vi "GetActiveFieldName.vi"(1 "protobuf index":i32) -> (0 "oneof field name":string)   [LabVIEW 2019, in "xnet-grpc_client.lvlib" / "nixnet_grpc_GetSubPropertySizeRequest_property_id_enum.lvclass"]
uses:
  nixnet_grpc_GetSubPropertySizeRequest_property_id_enum.lvclass
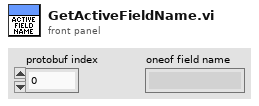
[diagram p1: front panel]
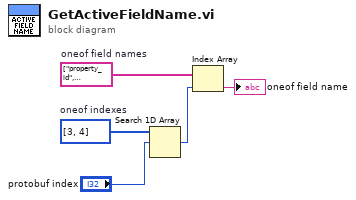
[diagram p0: block diagram]
diagram:
  w5 = string[] ["property_id", "property_id_raw"]  # oneof field names
  w4 = i32[] [3, 4]  # oneof indexes
  n1 = Search 1D Array(1D array=w4, element="protobuf index") -> (index of element=w2:i32)  [unwired: 1 in]
  n2 = Index Array(array=w5, index=w2) -> (element=→"oneof field name":string)
